vi "Convert property node font to graphics font.vi"(1 "String:Text:Font:All Elements font cluster":T1 caption="String:Text:Schriftart:Alle Elemente des Schriftartencluster") -> (0 "Get Text Rect font cluster":T2 caption="Schriftartencluster vom Textrechteck holen")   [LabVIEW 2009]
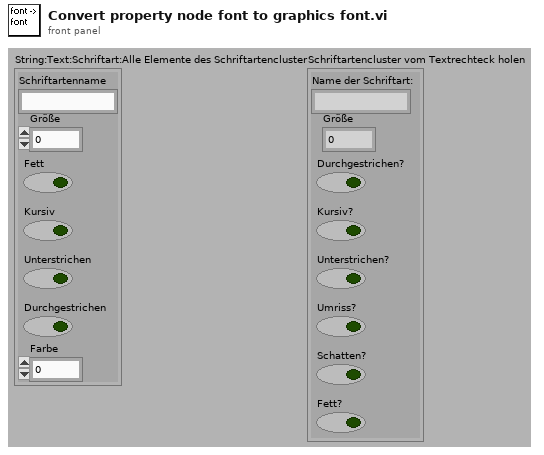
[diagram p1: front panel]
types:
  T1 = cluster{"Font Name":string, "Size":u16, "Bold":bool, "Italic":bool, "Underline":bool, "Strikeout":bool, "Color":u32}
  T2 = cluster{"Font Name:":string, "Size":i16, "Strikeout?":bool, "Italic?":bool, "Underline?":bool, "Outline?":bool, "Shadow?":bool, "Bold?":bool}
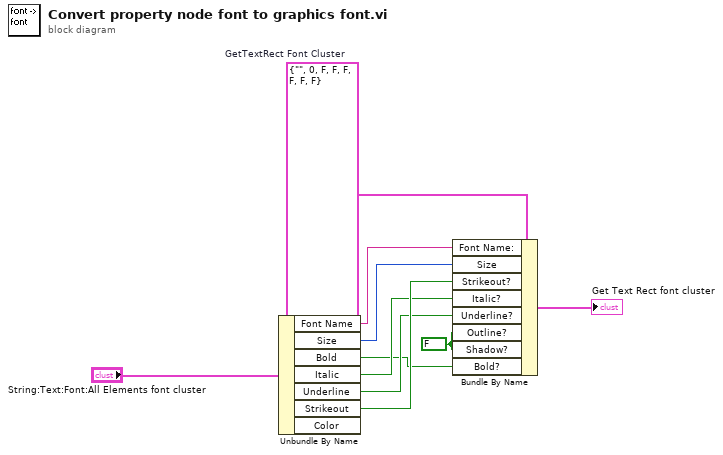
[diagram p0: block diagram]
diagram:
  w9 = FALSE ("Shadow?")
  w2 = T2 {"Font Name:"="", "Size"=0, "Strikeout?"=FALSE, "Italic?"=FALSE, "Underline?"=FALSE, "Outline?"=FALSE, "Shadow?"=FALSE, "Bold?"=FALSE}  # GetTextRect Font Cluster
  n1 = Unbundle By Name("String:Text:Font:All Elements font cluster") -> ("Font Name"=w3:string, "Size"=w4:u16, "Bold"=w5:bool, "Italic"=w6:bool, "Underline"=w7:bool, "Strikeout"=w8:bool)  [unwired: 1 out]
  n2 = Bundle By Name(cluster=w2, "Font Name:"=w3, "Size"=w4, "Strikeout?"=w8, "Italic?"=w6, "Underline?"=w7, "Outline?"=w9, "Shadow?"=w9, "Bold?"=w5) -> (→"Get Text Rect font cluster":T2)
